vi "Output Panel.vi"(8 "error in (no error)":errorcluster, 9 "Project In":refnum<class "Project.lvclass">, 11 "Step in":refnum<class "Step.lvclass">=refnum) -> (0 "error out":errorcluster, 3 "Step out":refnum<class "Step.lvclass">)   [LabVIEW 2015, in "OutputUI.lvclass"]
uses:
  OutputUI.lvclass
  Step.lvclass
  CallVIStep.lvclass
  Project.lvclass
  SerializableObject/CONFIGURE_UI_STATE.ctl
  Step/STEP_OUTPUT.ctl
  Step/OUTPUT_DATA_TYPE.ctl
  OUTPUT_CHECK_TYPE.ctl
  Step/OUTPUT_VALUE_TYPE.ctl
  Editor/Editor.lvclass
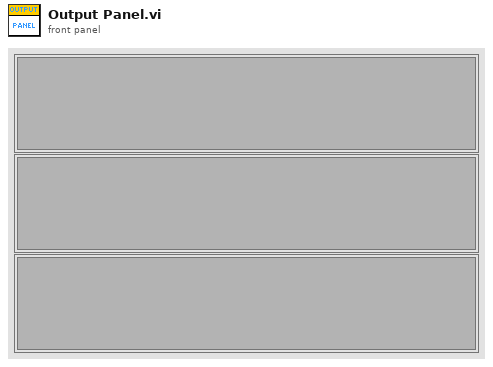
[diagram p1: front panel]
types:
  T1 = typedef "Editor.lvclass/CONFIGURE_UI_STATE.ctl" = enum16{"UI_LOOP", "INIT", "END", "CHANGE_PANEL"}
  T2 = typedef "Step.lvclass/STEP_OUTPUT.ctl" = cluster{"Label":string, "Name":string, "Data Type":T3, "Check Type":T4, "String Limit":string, "Lower Limit":dbl, "Upper Limit":dbl, "Boolean Limit":bool, "Ignore Case":bool, "Variable Name 1":string, "Limit Value Type 1":T5, "Variable Name 2":string, "Limit Value Type 2":T5}
  T3 = typedef "Step.lvclass/OUTPUT_DATA_TYPE.ctl" = enum16{"Boolean", "String", "Numeric", "Other"}
  T4 = typedef "Step.lvclass/OUTPUT_CHECK_TYPE.ctl" = enum16{"INVALID", "DO_NOT_CHECK", "RECORD", "VARIABLE", "EQUAL", "NOT_EQUAL", "STR_CONTAINS", "STR_START_WITH", "STR_END_WITH", "STR_REGEX_MATCH", "NUM_GT", "NUM_LT", "NUM_GE", "NUM_LE", "NUM_RANGE", "NUM_RANGE_BDY"}
  T5 = typedef "Step.lvclass/OUTPUT_VALUE_TYPE.ctl" = enum16{"Constant", "Variable"}
  T6 = typedef "LVRectTypeDef.ctl" = cluster{"Left":i16, "Top":i16, "Right":i16, "Bottom":i16}
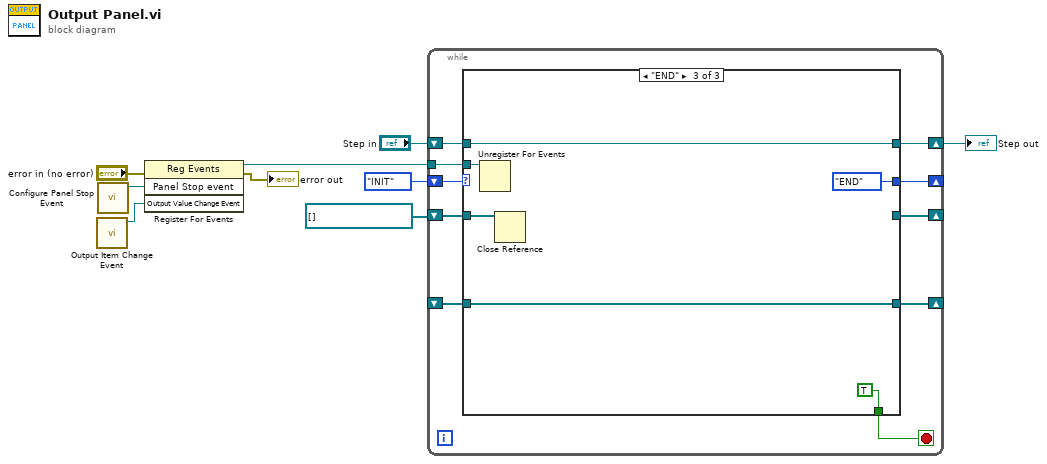
[diagram p0: block diagram]
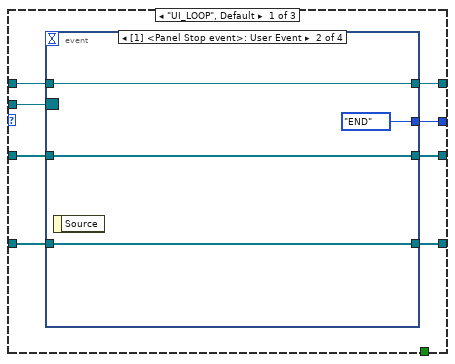
[diagram p2: hidden frame]
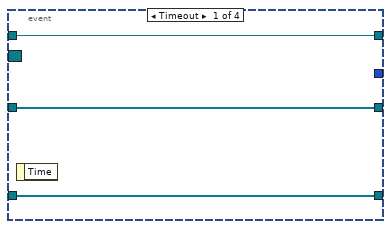
[diagram p3: hidden frame]
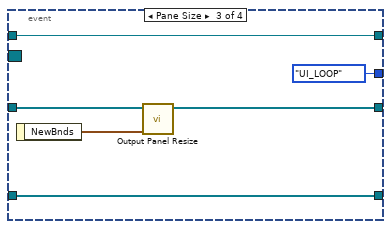
[diagram p4: hidden frame]
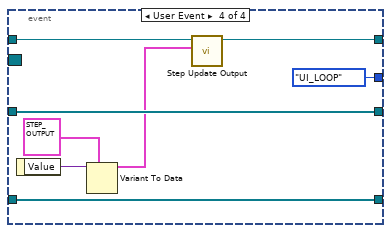
[diagram p5: hidden frame]
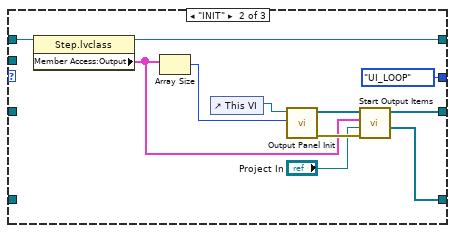
[diagram p6: hidden frame]
diagram:
  n1 = call "Output Item Change Event.vi"() -> ("Output Value Change Event"=w1:refnum<user-event>)  [unwired: 11 in]
  n2 = call "Configure Panel Stop Event.vi"() -> ("Panel Stop event"=w7:refnum<user-event>)  [unwired: 11 in]
  n3 = register-events(error in="error in (no error)", w7, w1) -> (reference out=w6:refnum<event-registration>, error out=→"error out":errorcluster)  [unwired: 1 in]
  n4 = while {
    shift-right: [w18] -> _
    shift-left: CONFIGURE_UI_STATE."INIT" -> [w19]
    shift-right: [w15] -> _
    shift-left: refnum<vi>[] [] -> [w16]
    tunnel: w6 -> [w14]
    shift-right: [w12] -> w4
    shift-left: "Step in" -> [w13]
    shift-right: [w11] -> _
    shift-left: _ -> [w10]
    stop <- w17 stop-if-true
    n5 = case shown="\"END\"" w19 {
      tunnel: [w27 CONFIGURE_UI_STATE."UI_LOOP" CONFIGURE_UI_STATE."END"] -> w18
      tunnel: [_ _ TRUE] -> w17
      tunnel: w16 -> [w26 _ w62]
      tunnel: [w25 w53 _] -> w15
      tunnel: w14 -> [w24 _ w63]
      tunnel: w13 -> [w21 w57 w61]
      tunnel: [w20 w56 w61] -> w12
      tunnel: [w22 w50 w60] -> w11
      tunnel: w10 -> [w23 _ w60]
      frame "UI_LOOP", Default {
        n6 = event shown="[1] <Panel Stop event>: User Event" {
          selector: w24 -> [_ _ _ _]
          dyn-events: _ -> [_ _ _ _]
          timeout: _ -> [_ _ _ _]
          tunnel: [_ CONFIGURE_UI_STATE."END" CONFIGURE_UI_STATE."UI_LOOP" CONFIGURE_UI_STATE."UI_LOOP"] -> w27
          tunnel: w26 -> [w30 w33 w39 w47]
          tunnel: [w30 w33 w38 w47] -> w25
          tunnel: [w29 w32 w37 w48] -> w22
          tunnel: w23 -> [w29 w32 w37 w48]
          tunnel: w21 -> [w28 w31 w35 w43]
          tunnel: [w28 w31 w35 w42] -> w20
          event Timeout {
            n7 = event-data() -> ()  [unwired: 1 in, 1 out]
          }
          event User Event {
            n8 = event-data() -> ()  [unwired: 1 in, 1 out]
          }
          event Pane Size {
            n9 = event-data() -> ("NewBnds"=w40:T6)  [unwired: 1 in]
            n10 = call "Output Panel Resize.vi"("NewBnds"=w40, "Item Panel in"=w39) -> ("Item Panel out"=w38:refnum<vi>[])  [unwired: 9 in]
          }
          event User Event {
            n11 = event-data() -> ("Value"=w45:variant)  [unwired: 1 in]
            n12 = Variant To Data(type=T2 {"Label"="", "Name"="", "Data Type"=enum."Boolean", "Check Type"=enum."INVALID", "String Limit"="", "Lower Limit"=0.0, "Upper Limit"=0.0, "Boolean Limit"=FALSE, "Ignore Case"=FALSE, "Variable Name 1"="", "Limit Value Type 1"=enum."Constant", "Variable Name 2"="", "Limit Value Type 2"=enum."Constant"} ("Output"), Variant=w45) -> (data=w41:T2)  [unwired: 1 in, 1 out]
            n13 = call "Step Update Output.vi"("Output in"=w41, "Step in"=w43) -> ("Step out"=w42:refnum<class "Step.lvclass">)  [unwired: 8 in, 1 out]
          }
        }
      }
      frame "INIT" {
        n14 = property class="Step.lvclass"(reference=w57) -> (reference out=w56:refnum<class "Step.lvclass">, "Member Access:Output"=w51:T2[])  [unwired: 1 in, 1 out]
        n15 = Array Size(array=w51) -> (size(s)=w55:i32)
        n16 = control-ref of="This VI"() -> (w58:refnum<vi>)
        n17 = call "Output Panel Init.vi"("Size"=w55, "VI in"=w58) -> ("error out"=w52:errorcluster, "Entry Panel out"=w54:refnum<vi>[])  [unwired: 8 in]
        n18 = call "Start Output Items.vi"("error in (no error)"=w52, "Project In"="Project In", "Output"=w51, "Item Panel in"=w54) -> ("Output Item VI Ref"=w50:refnum<vi>[], "Item Panel out"=w53:refnum<vi>[])  [unwired: 5 in, 1 out]
      }
      frame "END" {
        n19 = Unregister For Events(event registration refnum=w63) -> ()  [unwired: 1 in, 1 out]
        n20 = Close Reference(reference=w62) -> ()  [unwired: 1 in, 1 out]
      }
    }
  }
  "Step out" <- w4
